vi "Open Lockin.vi"(8 "error in (no error)":errorcluster, 10 "Lockin Address":string, 11 "MeasurementSMO in":refnum<class "MeasurementSMO.lvclass">) -> (0 "error out":errorcluster, 1 "Connected?":bool, 2 "ACK":string, 3 "MeasurementSMO out":refnum<class "MeasurementSMO.lvclass">)   [LabVIEW 2019, in "MeasurementSMO.lvclass"]
uses:
  MeasurementSMO.lvclass
  MeasurementSMO.lvclass/MeasurementSMO.ctl
  3a67aca2-1274-45bf-ad5a-6abfc6afcaa8.vi
  3a67aca2-1274-45bf-ad5a-6abfc6afcaa8.vi/ff40df25-0e41-4205-825d-56c19dc320b6.vi
  <userlib>/LevyLab/Lockin-Multichannel/Instrument.Lockin/Instrument.Lockin.lvclass
  C:/Program Files (x86)/National Instruments/LabVIEW 2019/user.lib/LevyLab/Instrument Framework/SMOs/Instrument/Instrument.lvclass
  <vilib>/Utility/Debug Log/Display.vi
  <userlib>/LevyLab/Instrument Framework/SMOs/Instrument/Instrument.lvclass
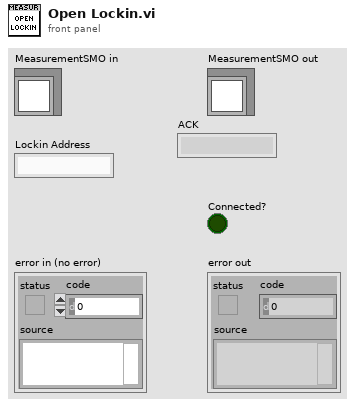
[diagram p1: front panel]
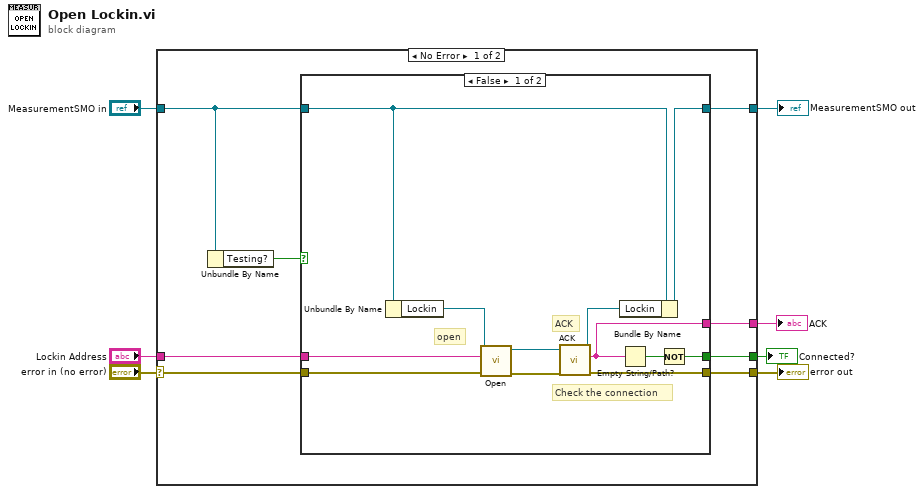
[diagram p0: block diagram]
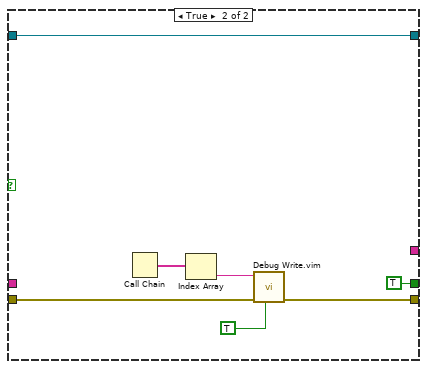
[diagram p2: hidden frame]
diagram:
  n1 = case shown="No Error" "error in (no error)" {
    selector: "error in (no error)" -> [w15 w36]
    tunnel: [w14 w36] -> w6
    tunnel: [w13 w35] -> w4
    tunnel: "MeasurementSMO in" -> [w11 w35]
    tunnel: "Lockin Address" -> [w12 _]
    tunnel: [w9 _] -> w2
    tunnel: [w8 _] -> w1
    frame No Error {
      n2 = Unbundle By Name(w11) -> ("Testing?"=w10:bool)
      n3 = case shown="False" w10 {
        tunnel: w15 -> [w23 w32]
        tunnel: [w20 w33] -> w14
        tunnel: [w26 w34] -> w13
        tunnel: w11 -> [w27 w34]
        tunnel: w12 -> [w22 _]
        tunnel: [w24 TRUE] -> w9
        tunnel: [w18 _] -> w8
        frame False {
          # "ACK"
          # "open"
          # "Check the connection"
          n4 = Unbundle By Name(w27) -> ("Lockin"=w21:refnum<class "Instrument.Lockin.lvclass">)
          n5 = call-dynamic "Open.vi"("error in (no error)"=w23, "address"=w22, "Instrument.Lockin in"=w21) -> ("error out"=w16:errorcluster, "Instrument.Lockin out"=w17:refnum<class "Instrument.Lockin.lvclass">)  [unwired: 7 in]
          n6 = call <userlib>:"ACK.vi"("error in (no error)"=w16, "Instrument in"=w17) -> ("error out"=w20:errorcluster, "ACK"=w18:string, "Instrument out"=w19:refnum<class "Instrument.Lockin.lvclass">)  [unwired: 7 in]
          n7 = Bundle By Name(cluster=w27, "Lockin"=w19) -> (w26:refnum<class "MeasurementSMO.lvclass">)
          n8 = Empty String/Path?(string/path=w18) -> (empty?=w25:bool)
          n9 = Not(x=w25) -> (.not. x?=w24:bool)
        }
        frame True {
          n10 = Call Chain() -> (call chain=w31:string[])
          n11 = Index Array(array=w31) -> (element=w30:string)  [unwired: 1 in]
          n12 = call "Debug Write.vim"("include timestamp? (F)"=TRUE, "error in (no error)"=w32, "value"=w30) -> ("error out"=w33:errorcluster)  [unwired: 8 in]
        }
      }
    }
    frame Error {
    }
  }
  "error out" <- w6
  "MeasurementSMO out" <- w4
  "Connected?" <- w2
  "ACK" <- w1
